vi "Logging Read All.vi"(4 "error in (no error)":errorcluster, 7 "LoggingDevRef":T5) -> (0 "error out":errorcluster, 2 "Log":T1[](array[typedef]), 3 "LoggingDevRef":T5)   [LabVIEW 2012, in "femtoRoboLib.lvlib"]
uses:
  femtoRoboLib.lvlib
  Controls/LoggingDevRef.ctl
  Controls/Log Entry - Full Block.ctl
  Controls/Log Entry.ctl
  Controls/Log Value Type.ctl
  Controls/Log Value Cluster.ctl
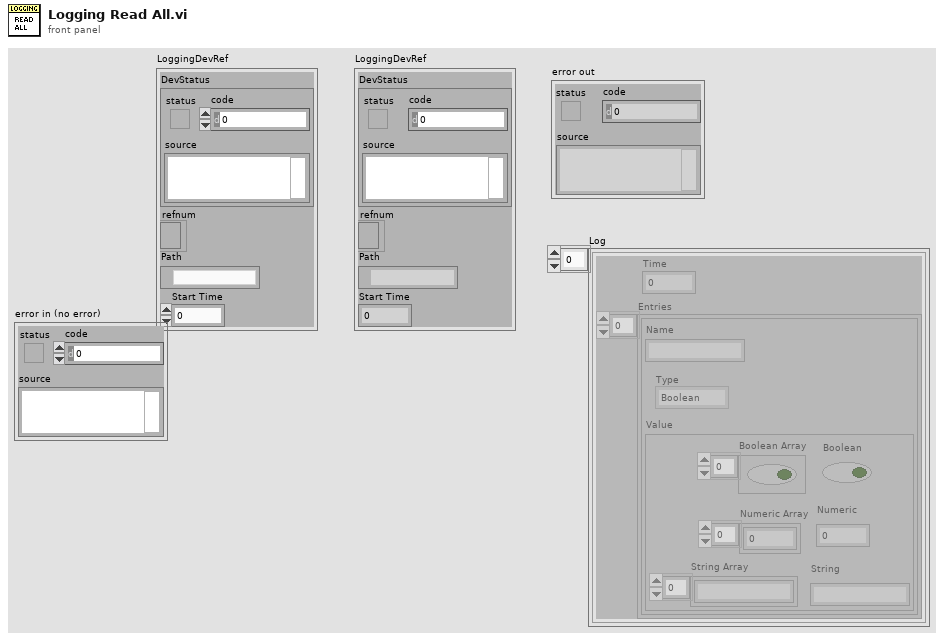
[diagram p1: front panel]
types:
  T1 = typedef "femtoRoboLib.lvlib/Log Entry - Full Block.ctl" = cluster{"Entries":T2[], "Time":u32}
  T2 = typedef "femtoRoboLib.lvlib/Log Entry.ctl" = cluster{"Name":string, "Type":T3, "Value":T4}
  T3 = typedef "femtoRoboLib.lvlib/Log Value Type.ctl" = enum16{"Boolean", "Numeric", "String", "Boolean Array", "Numeric Array", "String Array"}
  T4 = typedef "femtoRoboLib.lvlib/Log Value Cluster.ctl" = cluster{"Boolean Array":bool[], "Boolean":bool, "Numeric Array":dbl[], "Numeric":dbl, "String Array":string[], "String":string}
  T5 = typedef "femtoRoboLib.lvlib/LoggingDevRef.ctl" = cluster{"DevStatus":errorcluster, "refnum":refnum<file>, "Path":path, "Start Time":u32}
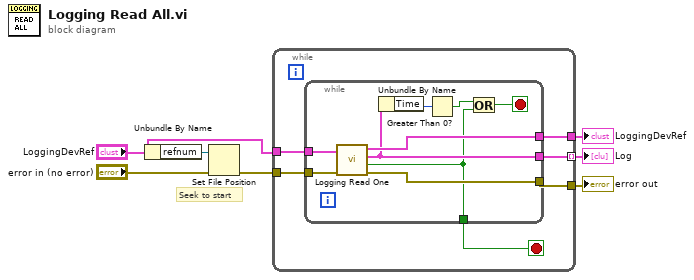
[diagram p0: block diagram]
diagram:
  # "Seek to start"
  n1 = Unbundle By Name("LoggingDevRef") -> ("refnum"=w6:refnum<file>)
  n2 = Set File Position(refnum=w6, error in="error in (no error)") -> (error out=w3:errorcluster)  [unwired: 2 in, 1 out]
  n3 = while {
    tunnel: [w9] -> w7 mode=indexing
    tunnel: "LoggingDevRef" -> [w13]
    tunnel: w3 -> [w12]
    tunnel: [w11] -> w1
    tunnel: [w10] -> w2
    stop <- w8 stop-if-true
    n4 = while {
      tunnel: w13 -> [w22]
      tunnel: w12 -> [w21]
      tunnel: [w20] -> w11
      tunnel: [w19] -> w10
      tunnel: [w18] -> w9
      tunnel: [w14] -> w8
      stop <- w15 stop-if-true
      n5 = call "Logging Read One.vi"("error in (no error)"=w21, "LoggingDevRef"=w22) -> ("error out"=w20:errorcluster, "EOF"=w14:bool, "Output"=w18:T1, "LoggingDevRef"=w19:T5)  [unwired: 2 in]
      n6 = Unbundle By Name(w18) -> ("Time"=w17:u32)
      n7 = Greater Than 0?(x=w17) -> (x > 0?=w16:bool)
      n8 = Or(x=w16, y=w14) -> (x .or. y?=w15:bool)
    }
  }
  "Log" <- w7
  "LoggingDevRef" <- w2
  "error out" <- w1
